vi "Serve.vi"(8 "error in (no error)":errorcluster, 11 "Table in":refnum<class "Table.lvclass">) -> (0 "error out":errorcluster, 3 "Table out":refnum<class "Table.lvclass">)   [LabVIEW 2023, in "Table.lvlib" / "Table.lvclass"]
uses:
  Table.lvclass
  Table.lvclass/Table.ctl
  Fork State.ctl
  Hungry State.ctl
  <vilib>/ActorFramework/Message Enqueuer/Message Enqueuer.lvclass/Message Enqueuer.ctl
  <vilib>/ActorFramework/Message Enqueuer/Enqueue.vi
  Philosopher/Philosopher Messages/Go to eating Msg/Eat.lvclass
  C:/Program Files (x86)/National Instruments/LabVIEW 2023/vi.lib/ActorFramework/Message/Message.lvclass
  <vilib>/ActorFramework/Message Priority Queue/Priority Enqueue.vi
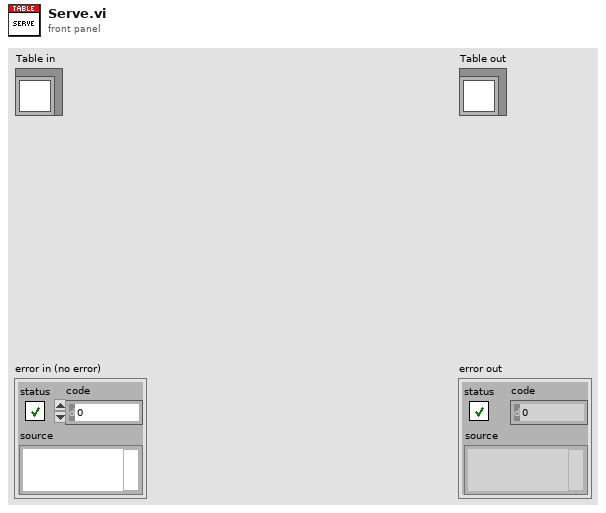
[diagram p1: front panel]
types:
  T1 = typedef "Table.lvlib/Table.lvclass/Hungry State.ctl" = enum16{"NO", "YES"}
  T2 = typedef "Table.lvlib/Table.lvclass/Fork State.ctl" = enum16{"FREE", "IN USE"}
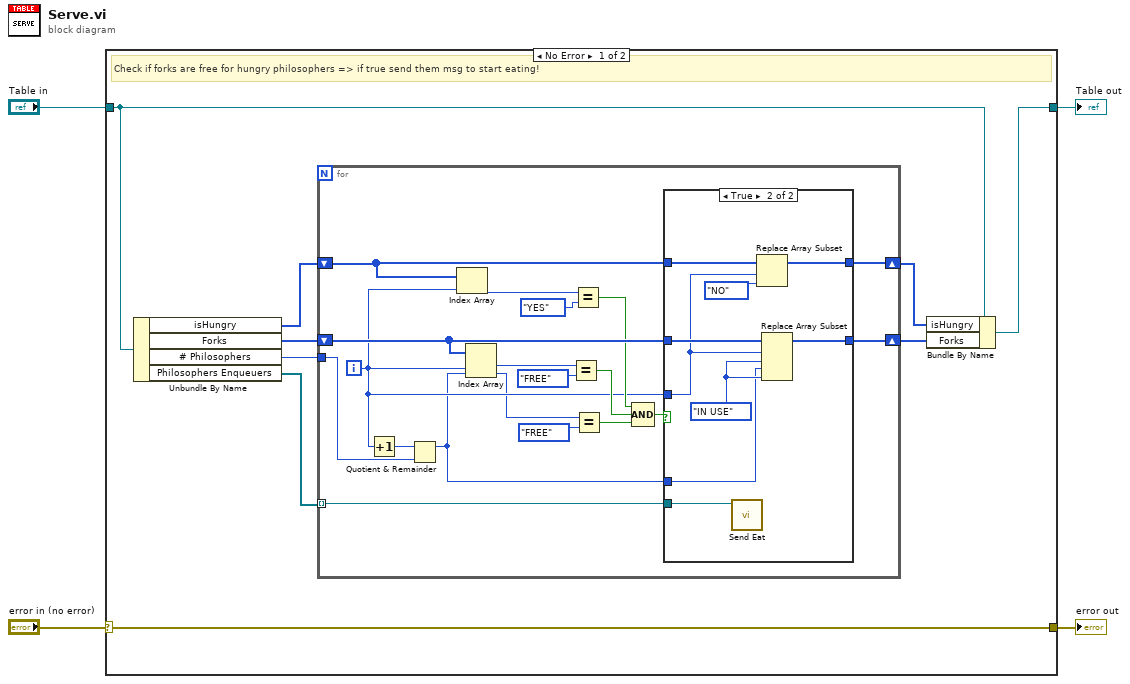
[diagram p0: block diagram]
diagram:
  n1 = case shown="No Error" "error in (no error)" {
    selector: "error in (no error)" -> [w13 w45]
    tunnel: [w13 w45] -> w3
    tunnel: [w9 w44] -> w1
    tunnel: "Table in" -> [w10 w44]
    frame No Error {
      # "Check if forks are free for hungry philosophers => if true send them msg to start eating!"
      n2 = Unbundle By Name(w10) -> ("isHungry"=w12:T1[], "Forks"=w11:T2[], "# Philosophers"=w5:i32, "Philosophers Enqueuers"=w7:refnum<class "Message Enqueuer.lvclass">[])
      n3 = for {
        tunnel: w5 -> [w31]
        shift-right: [w23] -> w8
        shift-left: w11 -> [w24]
        tunnel: w7 -> [w22] mode=indexing
        shift-right: [w17] -> w6
        shift-left: w12 -> [w18]
        i -> [w16]
        n4 = Increment(x=w16) -> (x+1=w32:i32)
        n5 = Quotient & Remainder(x=w32, y=w31) -> (x-y*floor(x/y)=w15:i32)  [unwired: 1 out]
        n6 = Index Array(array=w18, index=w16) -> (element=w21:T1)
        n7 = Index Array(array=w24, index #1=w16, index #2=w15) -> (element #1=w30:T2, element #2=w14:T2)
        n8 = Equal?(x=w30, y=Fork_State."FREE") -> (x = y?=w26:bool)
        n9 = Equal?(x=w21, y=Hungry_State."YES") -> (x = y?=w19:bool)
        n10 = Equal?(x=w14, y=Fork_State."FREE") -> (x = y?=w27:bool)
        n11 = Compound Arithmetic op=AND(w19, w26, w27) -> (w25:bool)
        n12 = case shown="True" w25 {
          tunnel: w24 -> [w34 w43]
          tunnel: w16 -> [_ w41]
          tunnel: w15 -> [_ w37]
          tunnel: [w34 w36] -> w23
          tunnel: w22 -> [_ w35]
          tunnel: w18 -> [w33 w42]
          tunnel: [w33 w39] -> w17
          frame False {
          }
          frame True {
            w38 = Fork_State."IN USE" ("y")
            n13 = call "Send Eat.vi"("Message Enqueuer"=w35) -> ()  [unwired: 9 in, 2 out]
            n14 = Replace Array Subset(array=w42, new element=Hungry_State."NO" ("new element/subarray"), index=w41) -> (w39:T1[])
            n15 = Replace Array Subset(array=w43, new element #1=w38, index #1=w41, new element #2=w38, index #2=w37) -> (w36:T2[])
          }
        }
      }
      n16 = Bundle By Name(cluster=w10, "isHungry"=w6, "Forks"=w8) -> (w9:refnum<class "Table.lvclass">)
    }
    frame Error {
    }
  }
  "error out" <- w3
  "Table out" <- w1
